vi "Configure Sequencer Dual Tone.vi"(6 "Level Ratio (0)":dbl, 7 "Frequency Offset (0Hz)":dbl format="%#.9p", 8 "error in (no error)":errorcluster, 9 "Source (1)":i32=1, 10 "Instance (1)":i32=1, 11 "VISA resource name":refnum<visa-resource-name>) -> (0 "error out":errorcluster, 3 "VISA resource name out":refnum<visa-resource-name>)   [LabVIEW 2020, in "Rohde&Schwarz CMXP GPRF.lvlib"]
doc: "Configures the dual tone sequencer.\n\nAttributes:\nRSCMXPGPRF_ATTR_SEQUENCER_FREQUENCY_OFFSET\nRSCMXPGPRF_ATTR_SEQUENCER_LEVEL_RATIO\n\nRemote-control commands:\nSOURce:GPRF:GEN<i>:SEQuencer:DTONe:OFRequency<source>\nSOURce:GPRF:GEN<i>:SEQuencer:DTONe:RATio"
uses:
  <instrlib>/Rohde&Schwarz CMXP GPRF/Rohde&Schwarz CMXP GPRF.lvlib
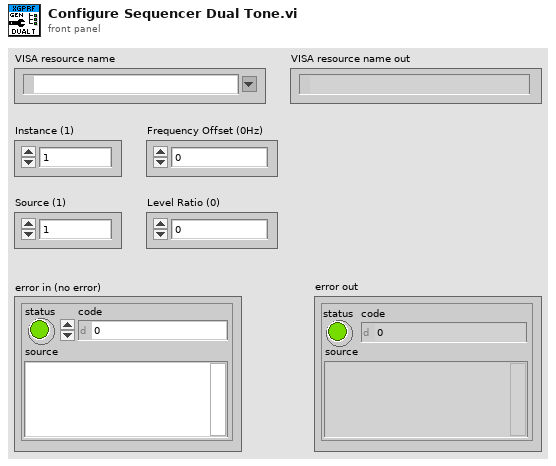
[diagram p1: front panel]
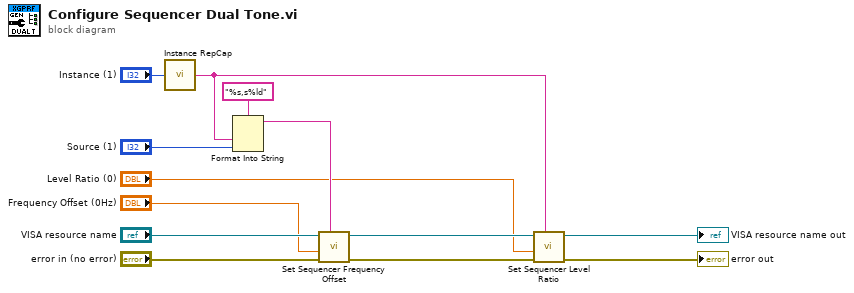
[diagram p0: block diagram]
diagram:
  n1 = call <instrlib>:"Instance RepCap.vi"("Instance in"="Instance (1)") -> ("Instance out"=w3:string)
  n2 = Format Into String(format string="%s,s%ld", w3, "Source (1)") -> (resulting string=w4:string)  [unwired: 2 in, 1 out]
  n3 = call "Set Sequencer Frequency Offset"("Repeated Capabilities"=w4, "error in (no error)"="error in (no error)", "Sequencer Frequency Offset (0.0)"="Frequency Offset (0Hz)", "instrument handle"="VISA resource name") -> ("error out"=w8:errorcluster, "instrument handle out"=w9:refnum<visa-resource-name>)  [unwired: 6 in]
  n4 = call "Set Sequencer Level Ratio"("Repeated Capabilities"=w3, "error in (no error)"=w8, "Sequencer Level Ratio (0.0)"="Level Ratio (0)", "instrument handle"=w9) -> ("error out"=→"error out":errorcluster, "instrument handle out"=→"VISA resource name out":refnum<visa-resource-name>)  [unwired: 6 in]
